vi "11120 UI.vi"(8 "error in (no error)":errorcluster, 11 "Node Ptr":T1 format="%.0x") -> (0 "error out":errorcluster)   [LabVIEW 2017, in "Modules.lvlib" / "11120.lvclass"]
uses:
  11120.lvclass
  <vilib>/NI Veristand/Custom Device API/Custom Device Item Ref.ctl
  RSI Module/SubPanel Command.ctl
  C:/Users/dbuck/Documents/GitHub/Scan-Engine-Custom-Device-Classes/Source/RemIO Module/RemIO Module.lvclass
  11120.lvclass/11120.ctl
  <vilib>/indcomecat/Remote IO/typedefs/REM-11120/channel number REM-11120.ctl
  RemIO Module/RemIO Module.lvclass
  <vilib>/indcomecat/Remote IO/NI ECAT Remote IO.lvlib
  <vilib>/NI Veristand/Custom Device API/Custom Device API.lvlib
  RSI Module/RSI Module.lvclass
panel:
  in  "Mounting Position":u8(ring) items=["Horizontal", "Vertical, bus coupler above", "Vertical, bus coupler below", "Lying"]
  out "_MountPositionlabel":string="Mounting Position"
  in  "Sensor Type":u8[](array[ring])=[1, 1, 1, 1] items=["K"=0, "J"=1, "E"=2, "R"=3, "S"=4, "T"=5, "B"=6, "N"=7, "U"=8, "L"=9, "C"=10, "W"=11, "HK"=12, "Cold junction"=15, "Linear voltage +-100 mV"=16, "Channel inactive"=31]
  out "_InputFilterllabel":string="Input Filter Time"
  in  "Resolution":u8[](array[ring])=[0, 0, 0, 0] items=["0.1 degrees Celsius (or 1 uV)", "1 degree Celsius (or 10 uV)", "0.1 degrees Fahrenheit", "1 degree Fahrenheit"]
  in  "Cold Junction Type":u8[](array[ring])=[0, 0, 0, 0] items=["Internal"=0, "Switched Off"=1, "External/Pt 100/Connector 1"=2, "External/Pt 100/Connector 2"=3, "Process data"=6]
  in  "Input Filter":u8[](array[ring])=[0, 0, 0, 0] items=["8.3 Hz", "10 Hz", "16.6 Hz", "25 Hz"]
  out "_Resolutionlabel":string="Resolution"
  out "_ColdJunctionlabel":string="Cold Junction Type"
  out "_Chan0Label":string="Channel 0"
  out "_Chan1Label":string="Channel 1"
  out "_Chan2Label":string="Channel 2"
  out "_Chan3Label":string="Channel 3"
  out "_SensorTypelabel":string="Sensor Type"
  in  "SubPanel Event":refnum<user-event>
  in  "Header":cluster{"Section Name":string}={"Section Name"="NI REM-11120 Settings"}
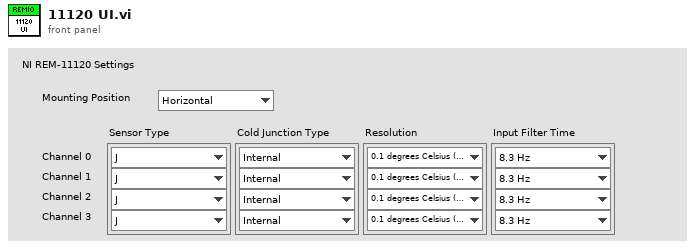
[diagram p1: front panel]
types:
  T1 = typedef "Custom Device API.lvlib/Custom Device Item Ref.ctl" = u64
  T2 = typedef "NI ECAT Remote IO.lvlib/mounting position REM-11120.ctl" = u8
  T3 = typedef "NI ECAT Remote IO.lvlib/channel number REM-11120.ctl" = u8
  T4 = typedef "NI ECAT Remote IO.lvlib/input filter time REM-11120.ctl" = u8
  T5 = typedef "NI ECAT Remote IO.lvlib/cold junction type REM-11120.ctl" = u8
  T6 = typedef "NI ECAT Remote IO.lvlib/resolution REM-11120.ctl" = u8
  T7 = typedef "NI ECAT Remote IO.lvlib/sensor type REM-11120.ctl" = u8
  T8 = cluster{"channel number":T3, "input filter time":T4, "cold junction type":T5, "resolution":T6, "sensor type":T7}[]
  T9 = typedef "Modules.lvlib/RSI Module.lvclass/SubPanel Command.ctl" = enum16{"Stop"}
  T10 = cluster{"channel number":T3, "Input Range 3":u8, "Input Filter 3":u8, "Mean Value 3":u8, "Mean Value 3":u8}
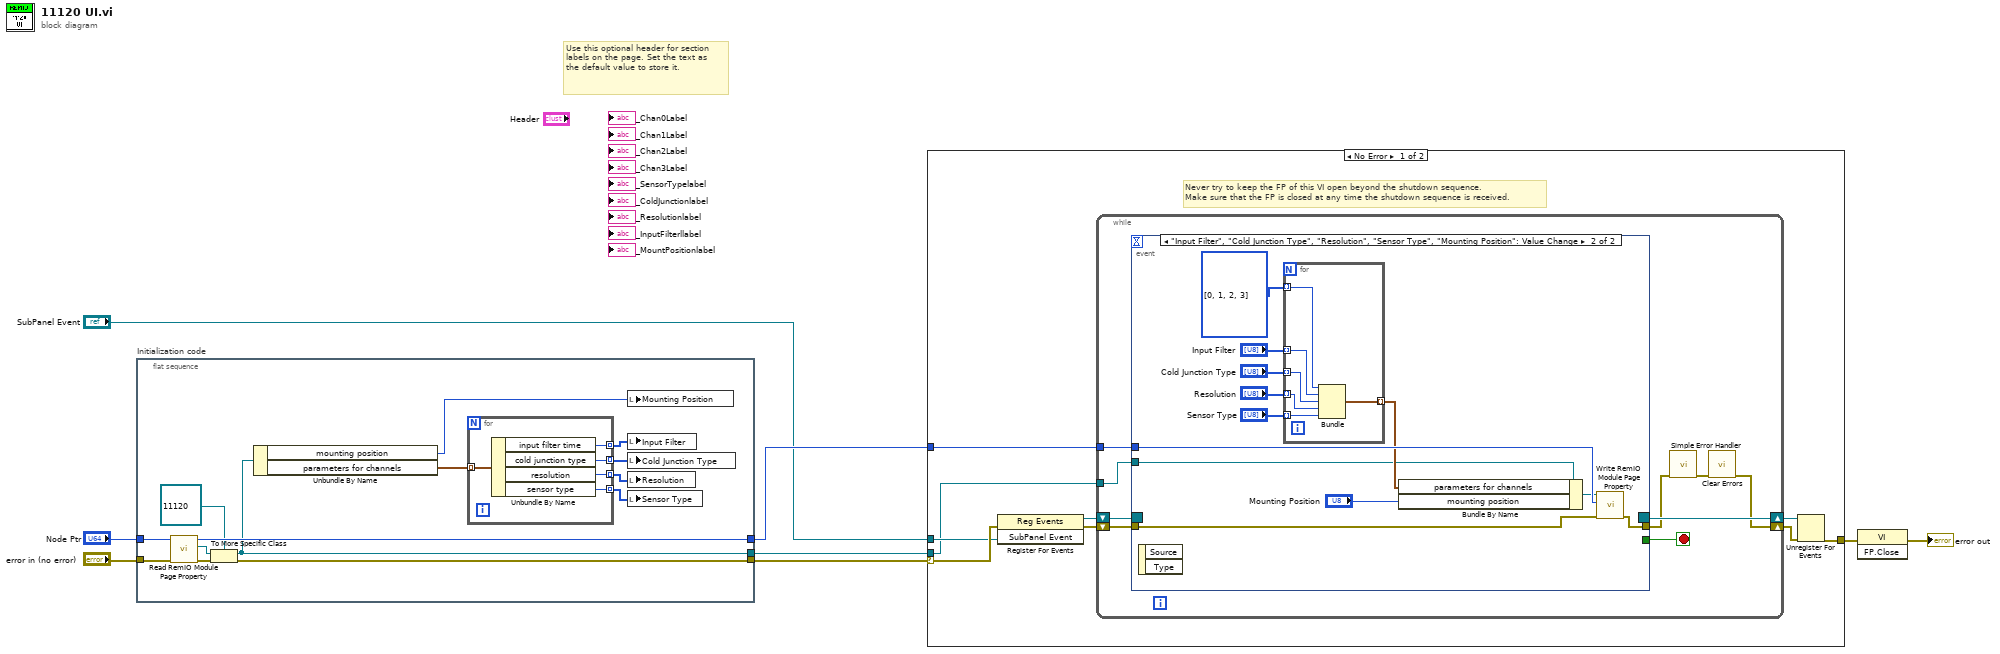
[diagram p0: block diagram]
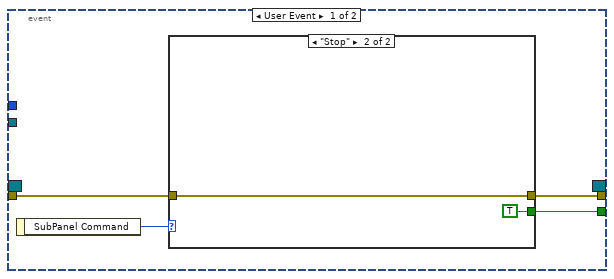
[diagram p2: hidden frame]
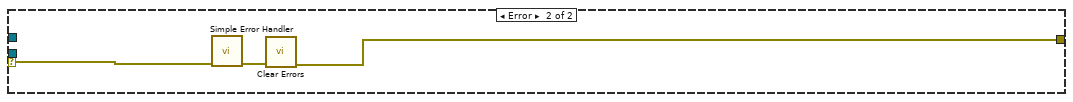
[diagram p4: hidden frame]
diagram:
  # "Use this optional header for section labels on the page. Set the text as the default value to store it."
  n1 = flat-sequence "Initialization code" {
    tunnel: "error in (no error)" -> [w21]
    tunnel: "Node Ptr" -> [w22]
    tunnel: [w17] -> w2
    tunnel: [w20] -> w5
    tunnel: [w14] -> w1
    frame #0 {
      n2 = call "Read RemIO Module Page Property.vi"("error in (no error)"=w21, "Node Ptr In"=w22) -> ("error out"=w19:errorcluster, "RemIO Module"=w18:refnum<class "RemIO Module.lvclass">, "Node Ptr Out"=w20:T1)  [unwired: 7 in]
      n3 = To More Specific Class(target class=refnum<class "11120.lvclass"> refnum ("Modules.lvlib:11120.lvclass"), reference=w18, error in=w19) -> (specific class reference=w14:refnum<class "11120.lvclass">, error out=w17:errorcluster)
      n4 = Unbundle By Name(w14) -> ("mounting position"=w9:T2, "parameters for channels"=w16:T8)
      n5 = for {
        tunnel: w16 -> [w24] mode=indexing
        tunnel: [w27] -> w12 mode=indexing
        tunnel: [w26] -> w13 mode=indexing
        tunnel: [w25] -> w11 mode=indexing
        tunnel: [w23] -> w10 mode=indexing
        n6 = Unbundle By Name(w24) -> ("input filter time"=w27:T4, "cold junction type"=w26:T5, "resolution"=w25:T6, "sensor type"=w23:T7)
      }
      n7 = local write "Mounting Position"(w9) -> ()
      n8 = local write "Input Filter"(w12) -> ()
      n9 = local write "Cold Junction Type"(w13) -> ()
      n10 = local write "Resolution"(w11) -> ()
      n11 = local write "Sensor Type"(w10) -> ()
    }
  }
  n12 = case shown="No Error" w2 {
    selector: w2 -> [w30 w73]
    tunnel: [w34 w71] -> w8
    tunnel: w5 -> [w31 _]
    tunnel: "SubPanel Event" -> [w29 _]
    tunnel: w1 -> [w28 _]
    frame No Error {
      # "Never try to keep the FP of this VI open beyond the shutdown sequence.\nMake sure that the FP is closed at any time the shutdown sequence is received."
      n13 = register-events(error in=w30, w29) -> (reference out=w32:refnum<event-registration>, error out=w33:errorcluster)  [unwired: 1 in]
      n14 = while {
        tunnel: w31 -> [w41]
        shift-right: [w38] -> w35
        shift-left: w33 -> [w44]
        shift-right: [w45] -> w36
        shift-left: w32 -> [w43]
        tunnel: w28 -> [w37]
        stop <- w42 stop-if-true
        n15 = event shown="[1] \"Input Filter\", \"Cold Junction Type\", \"Resolution\", \"Sensor Type\", \"Mounting Position\": Value Change" {
          selector: w43 -> [_ _]
          dyn-events: [_ _] -> w45
          timeout: _ -> [_ _]
          tunnel: w44 -> [w48 w63]
          tunnel: [w46 _] -> w42
          tunnel: [w47 w62] -> w40
          tunnel: w41 -> [_ w64]
          tunnel: w37 -> [_ w55]
          event User Event {
            n16 = event-data() -> ("SubPanel Command"=w49:T9)  [unwired: 1 out]
            n17 = case shown="\"Stop\"" w49 {
              tunnel: w48 -> [w50 w51]
              tunnel: [w50 w51] -> w47
              tunnel: [_ TRUE] -> w46
              frame Default {
              }
              frame "Stop" {
              }
            }
          }
          event "Input Filter", "Cold Junction Type", "Resolution", "Sensor Type", "Mounting Position": Value Change {
            w61 = T3[] [0, 1, 2, 3] items=["TC0", "TC1", "TC2", "TC3"]
            n18 = event-data() -> ()  [unwired: 3 out]
            n19 = for {
              tunnel: w61 -> [w70] mode=indexing
              tunnel: [w69] -> w60 mode=indexing
              tunnel: "Sensor Type" -> [w68] mode=indexing
              tunnel: "Resolution" -> [w67] mode=indexing
              tunnel: "Cold Junction Type" -> [w65] mode=indexing
              tunnel: "Input Filter" -> [w66] mode=indexing
              n20 = Bundle("channel number"=w70, "Input Range 3"=w66, "Input Filter 3"=w65, "Mean Value 3"=w67, "Mean Value 3"=w68) -> (w69:T10)  [unwired: 1 in]
            }
            n21 = Bundle By Name(cluster=w55, "parameters for channels"=w60, "mounting position"="Mounting Position") -> (w54:refnum<class "11120.lvclass">)
            n22 = call "Write RemIO Module Page Property.vi"("error in (no error)"=w63, "Node Ptr In"=w64, "RemIO Module"=w54) -> ("error out"=w62:errorcluster)  [unwired: 6 in, 2 out]
          }
        }
        n23 = call <vilib>:"Simple Error Handler.vi"("error in (no error)"=w40) -> ("error out"=w39:errorcluster)  [unwired: 1 in, 7 out]
        n24 = call <vilib>:"Clear Errors.vi"("error in (no error)"=w39) -> ("error out"=w38:errorcluster)  [unwired: 1 in, 5 out]
      }
      n25 = Unregister For Events(event registration refnum=w36, error in=w35) -> (error out=w34:errorcluster)
    }
    frame Error {
      n26 = call <vilib>:"Simple Error Handler.vi"("error in (no error)"=w73) -> ("error out"=w72:errorcluster)  [unwired: 1 in, 7 out]
      n27 = call <vilib>:"Clear Errors.vi"("error in (no error)"=w72) -> ("error out"=w71:errorcluster)  [unwired: 1 in, 5 out]
    }
  }
  n28 = invoke class="VI" method="FP.Close"(error in=w8) -> (error out=→"error out":errorcluster)  [unwired: 2 in, 2 out]
